vi "Value.vi"(11 "ElementsValue in":refnum<class "ElementsValue.lvclass">) -> (2 "Value":T1)   [LabVIEW 2020, in "Futures-Examples.lvlib" / "ElementsValue.lvclass"]
uses:
  ElementsValue.lvclass
  ElementsValue.lvclass/ElementsValue.ctl
  Some Fancy Data.ctl
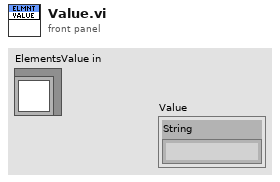
[diagram p1: front panel]
types:
  T1 = typedef "Futures-Examples.lvlib/ElementsValue.lvclass/Some Fancy Data.ctl" = cluster{"String":string}
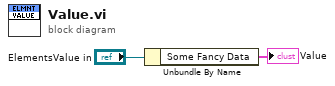
[diagram p0: block diagram]
diagram:
  n1 = Unbundle By Name("ElementsValue in") -> ("Some Fancy Data"=→"Value":T1)
